vi "drive_details.vi"(11 "Mission in":refnum<class "Mission.lvclass">) -> (1 "Drive Location":T1 {"North" format="%#_10f"; "East" format="%#_8f"}, 2 "Tolerance (m)":dbl, 3 "Mission out":refnum<class "Mission.lvclass">)   [LabVIEW 2011, in "Mission.lvclass"]
uses:
  Mission.lvclass
  2 Typedefs/UTM Location.ctl
  Mission.lvclass/Mission.ctl
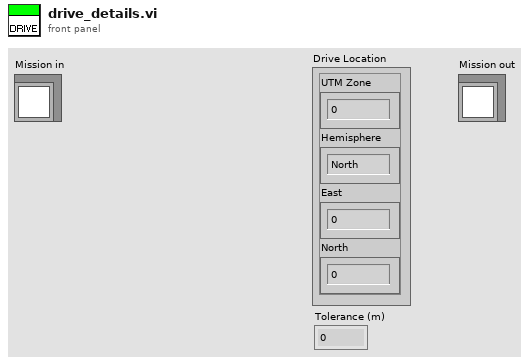
[diagram p1: front panel]
types:
  T1 = typedef "UTM Location.ctl" = cluster{"UTM Zone":dbl, "Hemisphere":enum16{"North", "South"}, "East":dbl, "North":dbl}
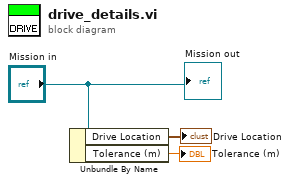
[diagram p0: block diagram]
diagram:
  n1 = Unbundle By Name("Mission in") -> ("Drive Location"=→"Drive Location":T1, "Tolerance (m)"=→"Tolerance (m)":dbl)
  "Mission out" <- "Mission in"
